vi "Begin.vi"(8 "error in (no error)":errorcluster, 11 "Comp Motors with Encoders in":refnum<class "Comp Motors with Encoders.lvclass">) -> (0 "error out":errorcluster, 3 "Comp Motors with Encoders out":refnum<class "Comp Motors with Encoders.lvclass">)   [LabVIEW 2014, in "Comp Motors with Encoders.lvlib" / "Comp Motors with Encoders.lvclass"]
uses:
  Comp Motors with Encoders.lvclass
  <vilib>/Rock Robotics/WPI/CAN/TalonSRX/WPI_CANTalonSRX_APIFeedbackSelect.ctl
  Comp Motors with Encoders.lvclass/Comp Motors with Encoders.ctl
  <vilib>/Rock Robotics/WPI/CAN/TalonSRX/WPI_CANTalonSRX_APIControlMode.ctl
  <vilib>/Rock Robotics/WPI/MotorControl/WPI_MotorControlOpenCANTalonSRX.vi
  Robot/Motor with Encoders/Motors with Encoders Class/Motors with Encoders.lvclass
panel:
  in  "Reverse Feedback Sensor":bool
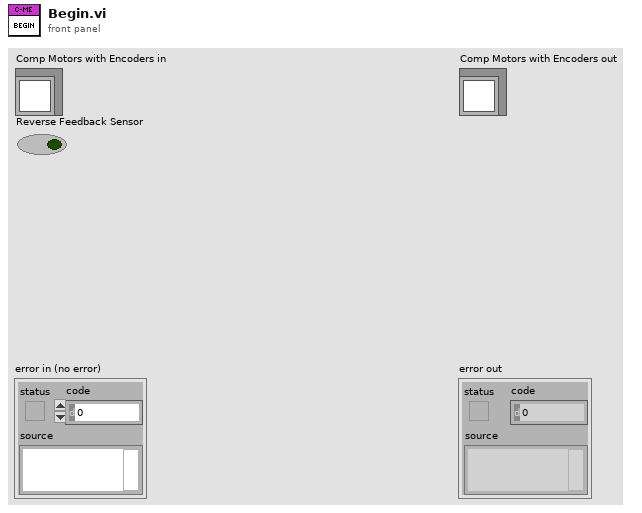
[diagram p1: front panel]
types:
  T1 = typedef "WPI_CANTalonSRX_APIFeedbackSelect.ctl" = enum16{"Digital Quadrature Encoder", "Analog Potentiometer", "Analog Encoder"}
  T2 = typedef "Motors with Encoders.lvlib/Motors with Encoders.lvclass/Motors with Encoders Config.ctl" = cluster{"Counts  Per Revolution":u32, "Invert Encoder Direction":bool, "Diameter of Revolution":dbl, "Max RPM":dbl, "Encoder Control":bool}
  T3 = typedef "WPI_CANTalonSRX_APIControlMode.ctl" = enum8{"Percent VBus", "Speed", "Position", "Slave", "Unchanged / Invalid"}
  T4 = typedef "Comp Motors with Encoders.lvlib/Comp Motors with Encoders.lvclass/Motor Controller Config.ctl" = cluster{"Device Number":u8, "Invert Motor":bool}
  T5 = typedef "Comp Motors with Encoders.lvlib/Comp Motors with Encoders.lvclass/Encoder Config.ctl" = cluster{"P":dbl, "D":dbl, "F":dbl, "I":dbl, "Reverse Feedback Sensor":bool, "Encoder Codes Per Rev":u16}
  T6 = typedef "WPI_MotorControlDeviceRef.ctl" = cluster{"DeviceStatus":errorcluster, "Type":T7, "PWM":cluster{"Controller":T8, "PWM Channel":T9, "DeadBand":T10}, "CAN":cluster{"Device Number":u8, "Control Mode":T11, "Semaphore":T12, "Max Vout":dbl, "TalonSRX Control Mode":T3}, "Invert":bool, "TransformRef":T13, "InvTransformRef":T13}
  T7 = typedef "WPI_MotorControlType.ctl" = enum16{"PWM", "CAN", "CANTalonSRX"}
  T8 = typedef "FPGA_TypedefDigitalModule.ctl" = enum16{"Controller 1"}
  T9 = typedef "FPGA_DIOPWMChannel.ctl" = enum8{"PWM 0", "PWM 1", "PWM 2", "PWM 3", "PWM 4", "PWM 5", "PWM 6", "PWM 7", "PWM 8", "PWM 9", "PWM MXP 0", "PWM MXP 1", "PWM MXP 2", "PWM MXP 3", "PWM MXP 4", "PWM MXP 5", "PWM MXP 6", "PWM MXP 7", "PWM MXP 8", "PWM MXP 9", "Invalid"}
  T10 = typedef "WPI_PWMDeadband.ctl" = cluster{"Name":string, "maxPositivePwm":i32, "minPositivePwm":i32, "centerPwm":i32, "maxNegativePwm":i32, "minNegativePwm":i32, "angularRange":u16}
  T11 = typedef "WPI_CANJaguar_ControlMode.ctl" = enum8{"Percent VBus", "Current", "Speed", "Position", "Voltage"}
  T12 = typedef "Semaphore RefNum" = refnum<k1>
  T13 = typedef "WPI_PWMTransform_ConPane.ctl" = refnum<vi>
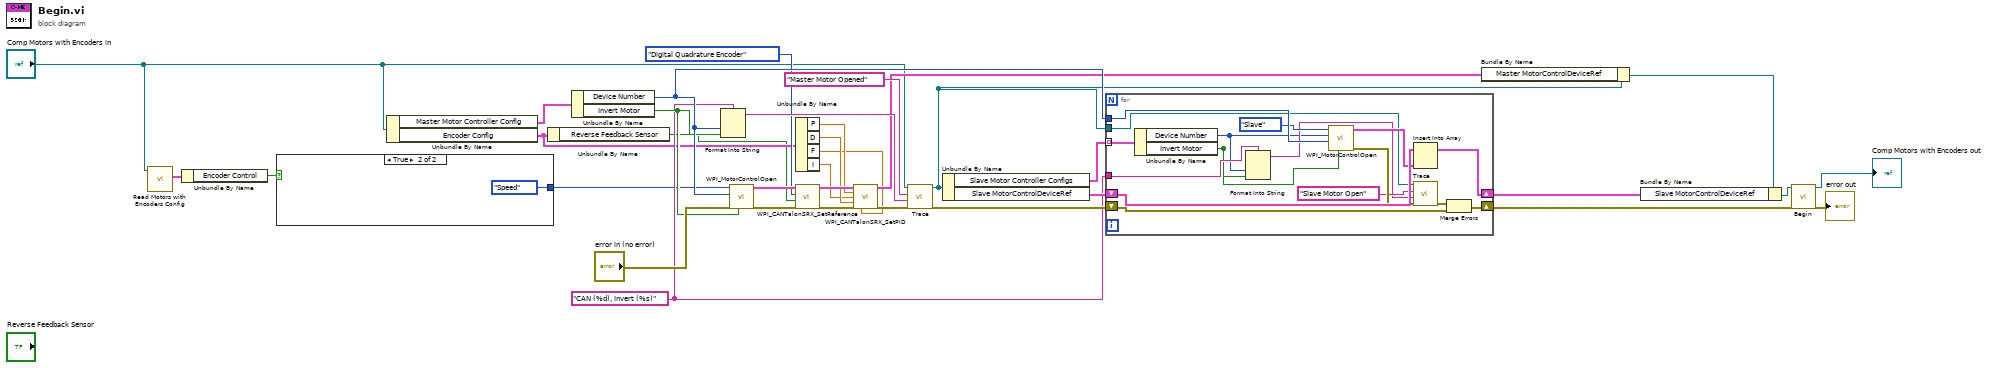
[diagram p0: block diagram]
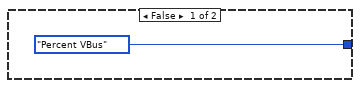
[diagram p2: hidden frame]
diagram:
  w18 = "CAN (%d), Invert (%s)" ("format string")
  n1 = call-dynamic "Read Motors with Encoders Config.vi"("Motors with Encoders in"="Comp Motors with Encoders in") -> ("Config"=w2:T2)  [unwired: 8 in, 2 out]
  n2 = Unbundle By Name(w2) -> ("Encoder Control"=w1:bool)
  n3 = case shown="True" w1 {
    tunnel: [WPI_CANTalonSRX_APIControlMode."Percent VBus" ("Control Mode") WPI_CANTalonSRX_APIControlMode."Speed" ("Control Mode")] -> w4
    frame False {
    }
    frame True {
    }
  }
  n4 = Unbundle By Name("Comp Motors with Encoders in") -> ("Master Motor Controller Config"=w32:T4, "Encoder Config"=w6:T5)
  n5 = Unbundle By Name(w6) -> ("Reverse Feedback Sensor"=w5:bool)
  n6 = Unbundle By Name(w32) -> ("Device Number"=w21:u8, "Invert Motor"=w20:bool)
  n7 = Format Into String(format string=w18, w21, w20) -> (resulting string=w22:string)  [unwired: 2 in, 1 out]
  n8 = call-poly <vilib>:"WPI_MotorControlOpen.vi"("Invert"=w20, "error in (no error)"="error in (no error)", "Device Number"=w21, "Control Mode"=w4) -> ("error out"=w16:errorcluster, "MotorControlDeviceRef"=w17:T6)  [unwired: 6 in]
  n9 = Unbundle By Name(w6) -> ("P"=w10:dbl, "D"=w9:dbl, "F"=w8:dbl, "I"=w7:dbl)
  n10 = call <vilib>:"WPI_CANTalonSRX_SetReference.vi"("error in (no error)"=w16, "Reverse Feedback Sensor"=w5, "Feedback Reference"=WPI_CANTalonSRX_APIFeedbackSelect."Digital Quadrature Encoder", "CAN Talon SRX Ref"=w17) -> ("error out"=w12:errorcluster, "CAN Talon SRX Ref Out"=w14:T6)  [unwired: 6 in]
  n11 = call <vilib>:"WPI_CANTalonSRX_SetPID.vi"("CAN Talon SRX Ref"=w14, "P"=w10, "I"=w7, "D"=w9, "error in (no error)"=w12, "F"=w8) -> ("CAN Talon SRX Ref Out"=w13:T6, "error out"=w11:errorcluster)  [unwired: 8 in]
  n12 = call-dynamic "Trace.vi"("error in (no error)"=w11, "System Message"=w22, "System Action"="Master Motor Opened", "System Actor in"="Comp Motors with Encoders in") -> ("error out"=w24:errorcluster, "System Actor out"=w19:refnum<class "Comp Motors with Encoders.lvclass">)  [unwired: 6 in]
  n13 = Unbundle By Name(w19) -> ("Slave Motor Controller Configs"=w28:T4[], "Slave MotorControlDeviceRef"=w27:T6[])
  n14 = for {
    tunnel: w28 -> [w52] mode=indexing
    tunnel: w21 -> [w51]
    shift-right: [w48] -> w25
    shift-left: w27 -> [w49]
    shift-right: [w46] -> w23
    shift-left: w24 -> [w47]
    tunnel: w19 -> [w44]
    tunnel: w18 -> [w41]
    n15 = Unbundle By Name(w52) -> ("Device Number"=w38:u8, "Invert Motor"=w37:bool)
    n16 = Format Into String(format string=w41, w38, w37) -> (resulting string=w39:string)  [unwired: 2 in, 1 out]
    n17 = call-poly <vilib>:"WPI_MotorControlOpen.vi"("Invert"=w37, "Master Device Number"=w51, "Device Number"=w38, "Control Mode"=WPI_CANTalonSRX_APIControlMode."Slave") -> ("error out"=w43:errorcluster, "MotorControlDeviceRef"=w45:T6)  [unwired: 6 in]
    n18 = Insert Into Array(array=w49, new element=w45) -> (w48:T6[])  [unwired: 1 in]
    n19 = call-dynamic "Trace.vi"("error in (no error)"=w43, "System Message"=w39, "System Action"="Slave Motor Open", "System Actor in"=w44) -> ("error out"=w42:errorcluster)  [unwired: 6 in, 1 out]
    n20 = Merge Errors(w42, w47) -> (w46:errorcluster)
  }
  n21 = Bundle By Name(cluster=w19, "Master MotorControlDeviceRef"=w13) -> (w31:refnum<class "Comp Motors with Encoders.lvclass">)
  n22 = Bundle By Name(cluster=w31, "Slave MotorControlDeviceRef"=w25) -> (w26:refnum<class "Comp Motors with Encoders.lvclass">)
  n23 = call-parent "Begin.vi"("error in (no error)"=w23, "System Actor in"=w26) -> ("error out"=→"error out":errorcluster, "System Actor out"=→"Comp Motors with Encoders out":refnum<class "Comp Motors with Encoders.lvclass">)  [unwired: 8 in]
